vi "Set Test Channel Move In Previous.vi"(8 "error in (no error)":errorcluster, 10 "Test Channel Move In Previous":bool, 11 "Abstract Test Channel Move In Previous Msg in":refnum<class "Abstract Test Channel Move In Previous Msg.lvclass">) -> (0 "error out":errorcluster, 3 "Abstract Test Channel Move In Previous Msg out":refnum<class "Abstract Test Channel Move In Previous Msg.lvclass">)   [LabVIEW 2013, in "Test Channel Model.lvlib" / "Abstract Test Channel Move In Previous Msg.lvclass"]
uses:
  Abstract Test Channel Move In Previous Msg.lvclass
  Abstract Test Channel Move In Previous Msg.lvclass/Abstract Test Channel Move In Previous Msg.ctl
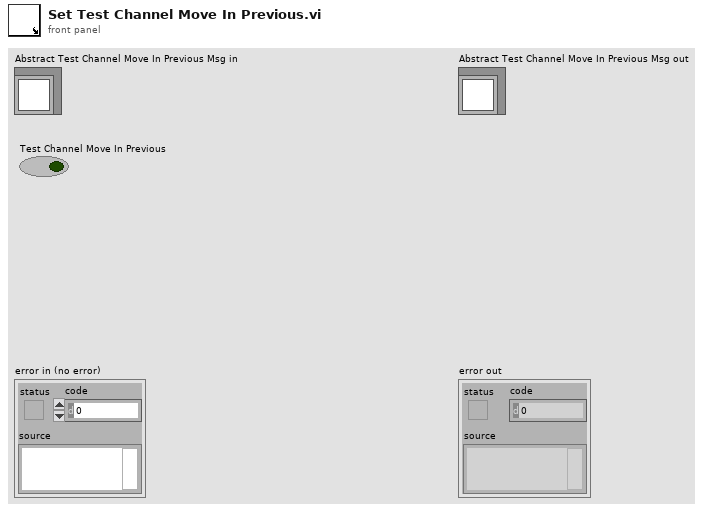
[diagram p1: front panel]
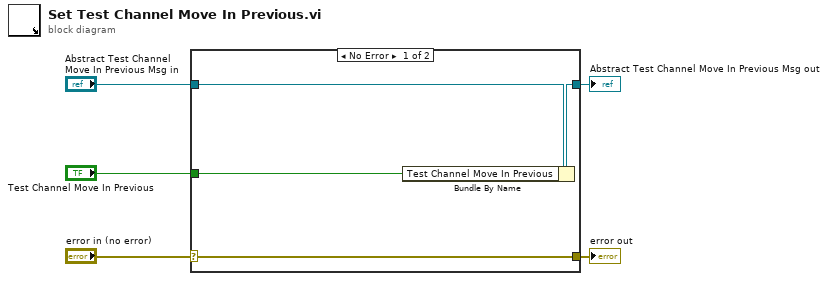
[diagram p0: block diagram]
diagram:
  n1 = case shown="No Error" "error in (no error)" {
    selector: "error in (no error)" -> [w9 w10]
    tunnel: [w9 w10] -> w4
    tunnel: [w7 w11] -> w2
    tunnel: "Abstract Test Channel Move In Previous Msg in" -> [w8 w11]
    tunnel: "Test Channel Move In Previous" -> [w6 _]
    frame No Error {
      n2 = Bundle By Name(cluster=w8, "Test Channel Move In Previous"=w6) -> (w7:refnum<class "Abstract Test Channel Move In Previous Msg.lvclass">)
    }
    frame Error {
    }
  }
  "error out" <- w4
  "Abstract Test Channel Move In Previous Msg out" <- w2
